vi "Set Disabled.vi"(8 "error in (no error)":errorcluster, 10 "Disabled":bool, 11 "GUI Element in":refnum<class "GUI Element.lvclass">) -> (0 "error out":errorcluster, 3 "GUI Element out":refnum<class "GUI Element.lvclass">)   [LabVIEW 2020, in "VolatusGUI.lvlib" / "GUI Element.lvclass"]
uses:
  GUI Element.lvclass
  GUI Element.lvclass/GUI Element.ctl
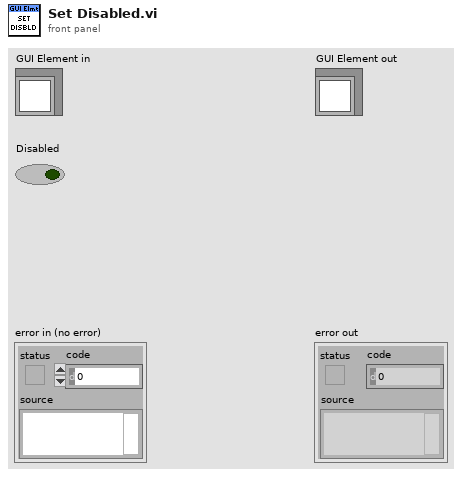
[diagram p1: front panel]
types:
  T1 = enum8{"Enabled", "Disabled", "Disabled and Grayed Out"}
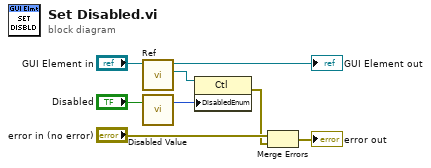
[diagram p0: block diagram]
diagram:
  n1 = call "Ref.vi"("GUI Element in"="GUI Element in") -> ("Ref"=w5:refnum<vi>, "GUI Element out"=→"GUI Element out":refnum<class "GUI Element.lvclass">)  [unwired: 9 in]
  n2 = call "Disabled Value.vi"("Disabled"="Disabled") -> ("Disabled Value"=w2:T1)  [unwired: 6 in]
  n3 = property class="Ctl"(reference=w5, "DisabledEnum"=w2) -> (error out=w3:errorcluster)  [unwired: 1 in, 1 out]
  n4 = Merge Errors("error in (no error)", w3) -> (→"error out":errorcluster)
